vi "Using Temperature.vi"() -> ()   [LabVIEW 2011]
doc: "This VI is designed to give experience using the Auto Tool. Refer to the LabVIEW Core I course for instructions."
panel:
  in  "Delay (sec)":dbl(slide) scale=0.0..10.0 scale format="%.1f"
  in  "Numeric":i32
  out "Temperature Graph":cluster{dbl[], dbl[]}(graph)
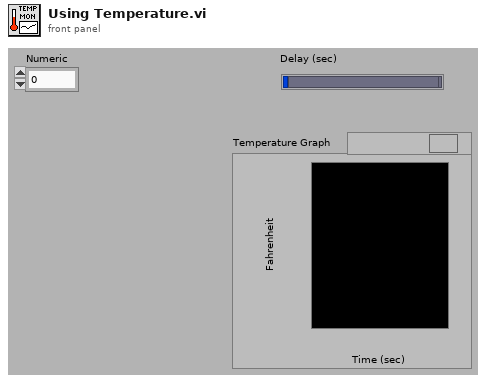
[diagram p1: front panel]
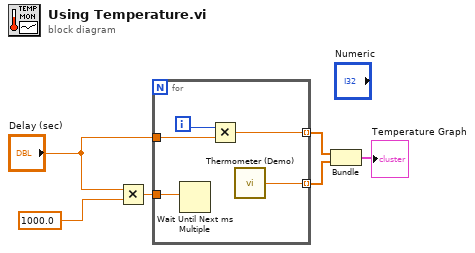
[diagram p0: block diagram]
diagram:
  n1 = Multiply(x="Delay (sec)", y=1000.0) -> (x*y=w5:dbl)
  n2 = for {
    tunnel: w5 -> [w11]
    tunnel: "Delay (sec)" -> [w9]
    tunnel: [w8] -> w4 mode=indexing
    tunnel: [w7] -> w3 mode=indexing
    i -> [w10]
    n3 = Wait Until Next ms Multiple(millisecond multiple=w11) -> ()  [unwired: 1 out]
    n4 = Multiply(x=w10, y=w9) -> (x*y=w8:dbl)
    n5 = call "Thermometer (Demo).vi"() -> ("Temperature"=w7:dbl)  [unwired: 1 in]
  }
  n6 = Bundle(w4, w3) -> (→"Temperature Graph":cluster{dbl[], dbl[]})  [unwired: 1 in]
